vi "OneButtonDialogWithTimeout.vi"(0 "Message text":string, 2 "Button text":string="OK", 3 "Timeout (s)":dbl=15.0 caption="Time Target (s)", 5 "Stopped":bool) -> ()   [LabVIEW 2016]
uses:
  user32.dll
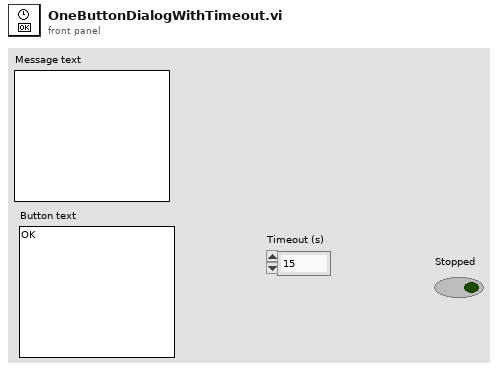
[diagram p1: front panel]
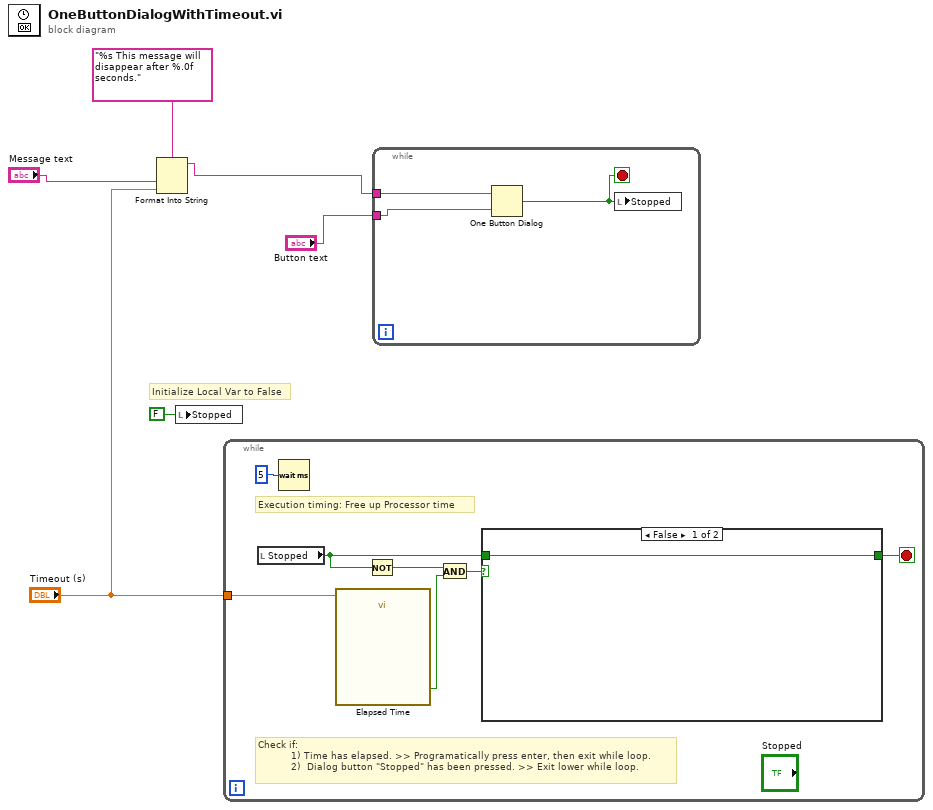
[diagram p0: block diagram]
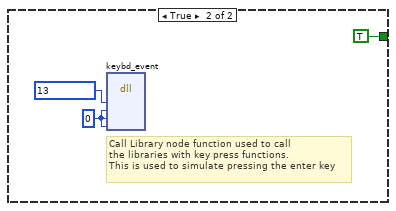
[diagram p2: hidden frame]
diagram:
  # "Initialize Local Var to False"
  n1 = Format Into String(format string="%s This message will disappear after %.0f seconds.", "Message text", "Timeout (s)") -> (resulting string=w4:string)  [unwired: 2 in, 1 out]
  n2 = local write "Stopped"(FALSE ("Stopped")) -> ()
  n3 = while {
    tunnel: "Timeout (s)" -> [w7]
    stop <- w13 stop-if-true
    # "Check if:\n           1) Time has elapsed. >> Programatically press enter, then exit while loop.\n           2)  Dialog button \"Stopped\" has been pressed. >> Exit lower while loop."
    # "Execution timing: Free up Processor time"
    n4 = local read "Stopped"() -> (w9:bool)
    n5 = Wait (ms)(milliseconds to wait=u32 5) -> ()  [unwired: 1 out]
    n6 = call "Elapsed Time"("Time Target (s)"=w7) -> ("Time has Elapsed"=w10:bool)  [unwired: 11 in, 7 out]
    n7 = Not(x=w9) -> (.not. x?=w11:bool)
    n8 = And(x=w11, y=w10) -> (x .and. y?=w12:bool)
    n9 = case shown="False" w12 {
      tunnel: [w14 TRUE] -> w13
      tunnel: w9 -> [w14 _]
      frame False {
      }
      frame True {
        w16 = u8 0 ("bScan")
        # "Call Library node function used to call \nthe libraries with key press functions. \nThis is used to simulate pressing the enter key"
        n10 = dll-call lib="user32.dll" fn="keybd_event"("bVk"=u8 13 ("Virtual Key"), "bScan"=w16, "dwFlags"=w16, "dwExtraInfo"=w16) -> ()  [unwired: 8 in, 2 out]
      }
    }
  }
  n11 = while {
    tunnel: w4 -> [w19]
    tunnel: "Button text" -> [w18]
    stop <- w20 stop-if-true
    n12 = One Button Dialog(message=w19, button name ("OK")=w18) -> (true=w20:bool)
    n13 = local write "Stopped"(w20) -> ()
  }
